vi "select_by_id.vi"(8 "Selection/Group":T3[](array[typedef]), 11 "Spots":T1[](array[typedef]) {"Amplitude Correction" step=0.1; "Line Trapping"."Phase Gradient" step=0.05; "Line Trapping"."Vector"."x" step=1e-06 format="%#_6p"; "Line Trapping"."Vector"."y" step=1e-06 format="%#_6p"; "Line Trapping"."Vector"."z" step=1e-06 format="%#_6p"; "NA Position"."r" step=1e-06; "NA Position"."y" step=1e-06; "NA Position"."x" step=1e-06; "Position"."z" step=1e-06; "Position"."y" step=1e-06; "Position"."x" step=1e-06; "Phase" step=0.7753; "Intensity" step=0.1}) -> (0 "Selection/Group Out":T3[](array[typedef]))   [LabVIEW 2010]
doc: "This VI pops up a dialog to allow the user to enter the ID of a spot or spots to select/deselect."
uses:
  selection_element.ctl
  spot.ctl
  line_trapping.ctl
  overlay_element.ctl
  red_tweezers_globals_INTERNAL.vi
panel:
  in  "Tab Control":enum32{"Spot", "Range", "Group"}(tab)=enum."Group"
  in  "ID":i32
  in  "to":i32
  in  "Range:":i32
  in  "Group ID":i32
  in  "Cancel":bool
  in  "OK Button":bool
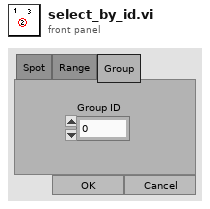
[diagram p1: front panel]
types:
  T1 = typedef "spot.ctl" = cluster{"Position":cluster{"x":dbl, "y":dbl, "z":dbl}, "Intensity":dbl, "Vortex Charge":i8, "Phase":dbl, "NA Position":cluster{"x":dbl, "y":dbl, "r":dbl}, "Line Trapping":T2, "Amplitude Correction":dbl}
  T2 = typedef "line_trapping.ctl" = cluster{"Vector":cluster{"x":dbl, "y":dbl, "z":dbl}, "Phase Gradient":dbl}
  T3 = typedef "selection_element.ctl" = cluster{"Group ID":i32, "Selected":bool}
  T4 = typedef "overlay_element.ctl" = cluster{"Tool":enum16{"Lines", "Oval", "Rectangle", "Text"}, "Points":cluster{"X":dbl, "Y":dbl}[], "Drawing Mode":u32, "Color":u32, "String":string}
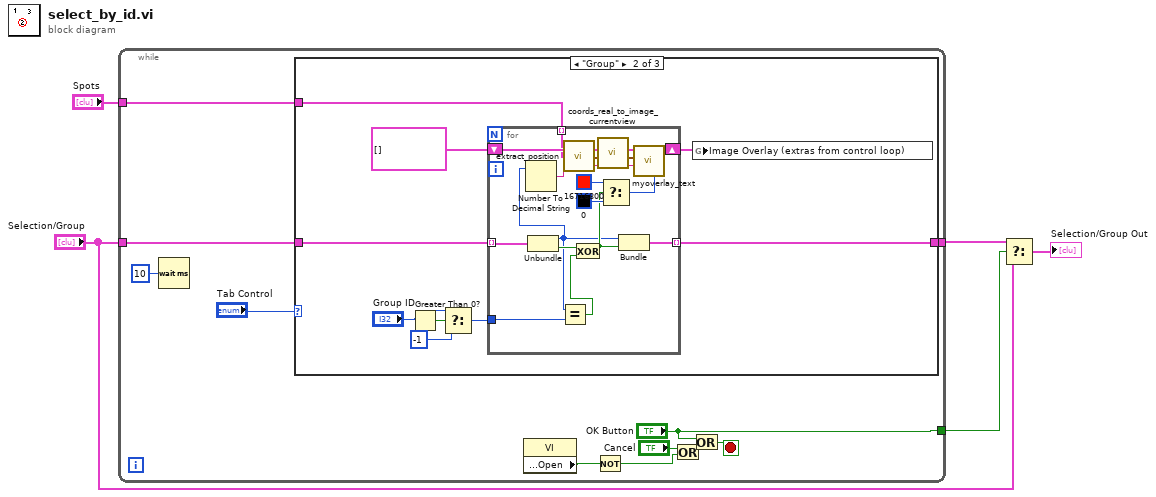
[diagram p0: block diagram]
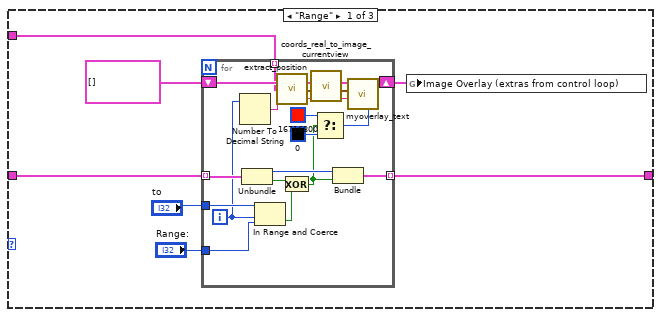
[diagram p2: hidden frame]
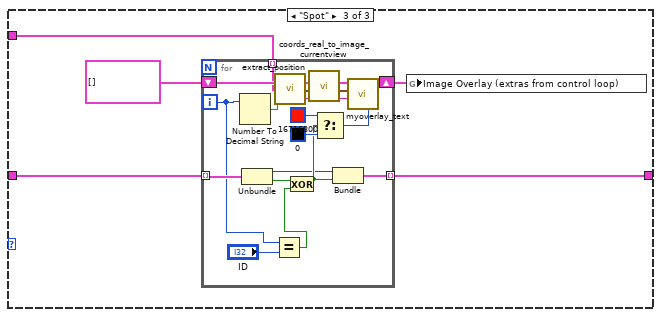
[diagram p3: hidden frame]
diagram:
  n1 = while {
    tunnel: "Spots" -> [w15]
    tunnel: "Selection/Group" -> [w14]
    tunnel: [w12] -> w4
    tunnel: ["OK Button"] -> w3
    stop <- w10 stop-if-true
    n2 = Wait (ms)(milliseconds to wait=u32 10) -> ()  [unwired: 1 out]
    n3 = case shown="\"Group\"" "Tab Control" {
      tunnel: w15 -> [w17 w46 w67]
      tunnel: w14 -> [w20 w49 w70]
      tunnel: [w18 w47 w68] -> w12
      frame "Range" {
        n4 = for {
          shift-right: [w30] -> w19
          shift-left: T4[] [] ("Overlay Elements In") -> [w41]
          tunnel: "Range:" -> [w40]
          tunnel: "to" -> [w39]
          tunnel: w20 -> [w38] mode=indexing
          tunnel: [w27] -> w18 mode=indexing
          tunnel: w17 -> [w25] mode=indexing
          i -> [w31]
          n5 = Number To Decimal String(number=w31) -> (decimal integer string=w32:string)  [unwired: 1 in]
          n6 = Unbundle(w38) -> ("Group ID"=w29:i32, "Selected"=w37:bool)
          n7 = In Range and Coerce(upper limit=w39, x=w31, lower limit=w40) -> (In Range?=w36:bool)  [unwired: 1 out]
          n8 = call "extract_position.vi"("Spot"=w25) -> ("Position"=w26:cluster{"x":dbl, "y":dbl, "z":dbl})
          n9 = Exclusive Or(1:w36, 2:w37) -> (0:w28:bool)
          n10 = call "coords_real_to_image_currentview.vi"("Position (real coords)"=w26) -> ("Position (pixels, relative to the top left of the image)"=w24:cluster{dbl, dbl})  [unwired: 7 in, 1 out]
          n11 = Select(t=u32 16716800 ("Color"), s=w28, f=u32 0 ("Color")) -> (s? t:f=w33:u32)
          n12 = Bundle("Group ID"=w29, w28) -> (w27:cluster{"Group ID":i32, bool})  [unwired: 1 in]
          n13 = call "myoverlay_text.vi"("Color"=w33, "String"=w32, "Centre Position (pixels on image)"=w24, "Overlay Elements In"=w41) -> ("Overlay Elements Out"=w30:T4[])  [unwired: 5 in]
        }
        n14 = global write "red_tweezers_globals_INTERNAL.vi" "Image Overlay (extras from control loop)"(w19) -> ()
      }
      frame "Group" {
        n15 = Greater Than 0?(x="Group ID") -> (x > 0?=w45:bool)
        n16 = Select(t="Group ID", s=w45, f=-1) -> (s? t:f=w42:i32)
        n17 = for {
          shift-right: [w59] -> w48
          shift-left: T4[] [] ("Overlay Elements In") -> [w66]
          tunnel: w49 -> [w65] mode=indexing
          tunnel: [w57] -> w47 mode=indexing
          tunnel: w46 -> [w53] mode=indexing
          tunnel: w42 -> [w52]
          n18 = Unbundle(w65) -> ("Group ID"=w56:i32, "Selected"=w64:bool)
          n19 = Number To Decimal String(number=w56) -> (decimal integer string=w60:string)  [unwired: 1 in]
          n20 = Equal?(x=w56, y=w52) -> (x = y?=w55:bool)
          n21 = call "extract_position.vi"("Spot"=w53) -> ("Position"=w54:cluster{"x":dbl, "y":dbl, "z":dbl})
          n22 = Exclusive Or(1:w55, 2:w64) -> (0:w58:bool)
          n23 = call "coords_real_to_image_currentview.vi"("Position (real coords)"=w54) -> ("Position (pixels, relative to the top left of the image)"=w51:cluster{dbl, dbl})  [unwired: 7 in, 1 out]
          n24 = Select(t=u32 16716800 ("Color"), s=w58, f=u32 0 ("Color")) -> (s? t:f=w61:u32)
          n25 = Bundle("Group ID"=w56, w58) -> (w57:cluster{"Group ID":i32, bool})  [unwired: 1 in]
          n26 = call "myoverlay_text.vi"("Color"=w61, "String"=w60, "Centre Position (pixels on image)"=w51, "Overlay Elements In"=w66) -> ("Overlay Elements Out"=w59:T4[])  [unwired: 5 in]
        }
        n27 = global write "red_tweezers_globals_INTERNAL.vi" "Image Overlay (extras from control loop)"(w48) -> ()
      }
      frame "Spot" {
        n28 = for {
          shift-right: [w82] -> w69
          shift-left: T4[] [] ("Overlay Elements In") -> [w75]
          tunnel: w70 -> [w88] mode=indexing
          tunnel: [w80] -> w68 mode=indexing
          tunnel: w67 -> [w74] mode=indexing
          i -> [w76]
          n29 = Number To Decimal String(number=w76) -> (decimal integer string=w83:string)  [unwired: 1 in]
          n30 = Unbundle(w88) -> ("Group ID"=w77:i32, "Selected"=w87:bool)
          n31 = Equal?(x=w76, y="ID") -> (x = y?=w79:bool)
          n32 = call "extract_position.vi"("Spot"=w74) -> ("Position"=w73:cluster{"x":dbl, "y":dbl, "z":dbl})
          n33 = Exclusive Or(1:w79, 2:w87) -> (0:w81:bool)
          n34 = call "coords_real_to_image_currentview.vi"("Position (real coords)"=w73) -> ("Position (pixels, relative to the top left of the image)"=w72:cluster{dbl, dbl})  [unwired: 7 in, 1 out]
          n35 = Select(t=u32 16716800 ("Color"), s=w81, f=u32 0 ("Color")) -> (s? t:f=w84:u32)
          n36 = Bundle("Group ID"=w77, w81) -> (w80:cluster{"Group ID":i32, bool})  [unwired: 1 in]
          n37 = call "myoverlay_text.vi"("Color"=w84, "String"=w83, "Centre Position (pixels on image)"=w72, "Overlay Elements In"=w75) -> ("Overlay Elements Out"=w82:T4[])  [unwired: 5 in]
        }
        n38 = global write "red_tweezers_globals_INTERNAL.vi" "Image Overlay (extras from control loop)"(w69) -> ()
      }
    }
    n39 = property class="VI"() -> ("Front Panel.Open"=w7:bool)  [unwired: 2 in, 2 out]
    n40 = Not(x=w7) -> (.not. x?=w6:bool)
    n41 = Or(x="Cancel", y=w6) -> (x .or. y?=w8:bool)
    n42 = Or(x="OK Button", y=w8) -> (x .or. y?=w10:bool)
  }
  n43 = Select(t=w4, s=w3, f="Selection/Group") -> (s? t:f=→"Selection/Group Out":T3[])
